vi "REPLACE.vi"(11 "jettl in":refnum<class "jettl.lvclass">) -> (2 "Destroy?":bool, 3 "jettl out":refnum<class "jettl.lvclass">)   [LabVIEW 2021, in "jettl.lvlib" / "jettl.lvclass"]
uses:
  jettl.lvclass
  C:/git/jettl/src/Actor/Actor/Actor.lvclass
  jettl.lvclass/jettl.ctl
  State/State/State.lvclass
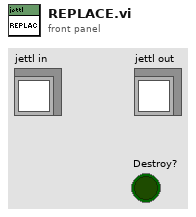
[diagram p1: front panel]
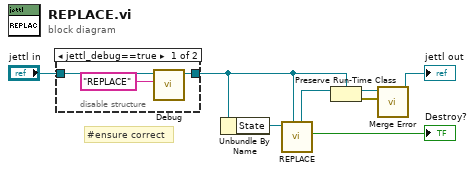
[diagram p0: block diagram]
diagram:
  # "#ensure correct"
  n1 = disable-structure shown="jettl_debug==true" {
    disable-tunnel: "jettl in" -> [w11 w12]
    disable-tunnel: [w10 w12] -> w1
    frame condition #0 (active) {
      n2 = call "Debug.vi"("Method"="REPLACE", "jettl in"=w11) -> ("jettl out"=w10:refnum<class "jettl.lvclass">)  [unwired: 9 in]
    }
    frame condition #1 {
    }
  }
  n3 = Unbundle By Name(w1) -> ("State"=w8:refnum<class "State.lvclass">)
  n4 = call-dynamic "REPLACE.vi"("Actor in"=w1, "State in"=w8) -> ("Destroy?"=→"Destroy?":bool, "Actor out"=w6:refnum<class "Actor.lvclass">)  [unwired: 8 in]
  n5 = Preserve Run-Time Class(object in=w6, 2:w1) -> (object out=w5:refnum<class "jettl.lvclass">, error out=w3:errorcluster)  [unwired: 1 in]
  n6 = call-dynamic "Merge Error.vi"("Error"=w3, "jettl in"=w5) -> ("jettl out"=→"jettl out":refnum<class "jettl.lvclass">)  [unwired: 9 in]
